vi "Ejer3_tabla.vi"() -> ()   [LabVIEW 2020]
panel:
  in  "stop":bool
  out "Table Indicador":string[][](table)
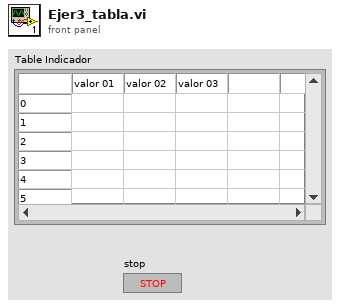
[diagram p1: front panel]
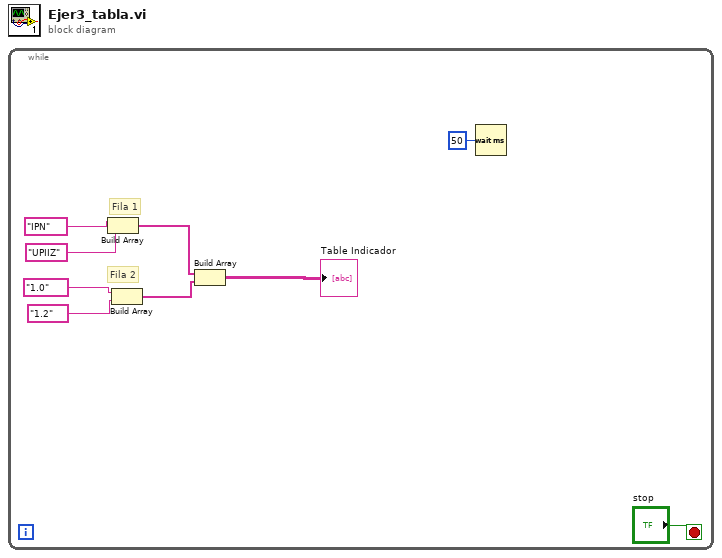
[diagram p0: block diagram]
diagram:
  n1 = while {
    stop <- "stop" stop-if-true
    # "Fila 2"
    # "Fila 1"
    n2 = Build Array("IPN", "UPIIZ") -> (w9:string[])
    n3 = Build Array("1.0", "1.2") -> (w8:string[])
    n4 = Build Array "Build Array"(w9, w8) -> (→"Table Indicador":string[][])
    n5 = Wait (ms)(milliseconds to wait=u32 50) -> ()  [unwired: 1 out]
  }
